vi "OneShotPulse.vi"(11 "Input":bool) -> (3 "Output":bool)   [LabVIEW 2016]
doc: "When the input goes true, the output goes true for one iteration.\nIt stays false until the input goes false and true again"
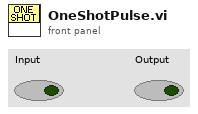
[diagram p1: front panel]
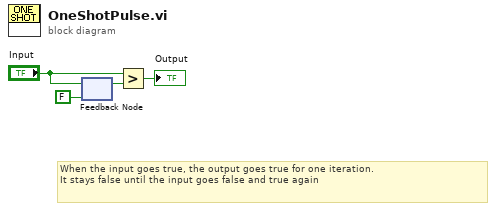
[diagram p0: block diagram]
diagram:
  # "When the input goes true, the output goes true for one iteration.\nIt stays false until the input goes false and true again"
  n1 = feedback-in #1("Input") -> ()
  n2 = feedback #1(FALSE ("Input")) -> (w4:bool)
  n3 = Greater?(x="Input", y=w4) -> (0:→"Output":bool)
